vi "measure.vi"(8 "error in (no error)":errorcluster, 10 "Measure":bool, 11 "handle":i32) -> (0 "error out":errorcluster, 3 "state":i32)   [LabVIEW 2018]
uses:
  <userlib>/Gigahertz-Optik/GOMDTR9600/GOMDTR9600.lvlib
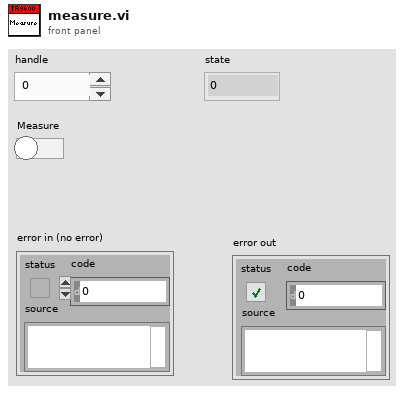
[diagram p1: front panel]
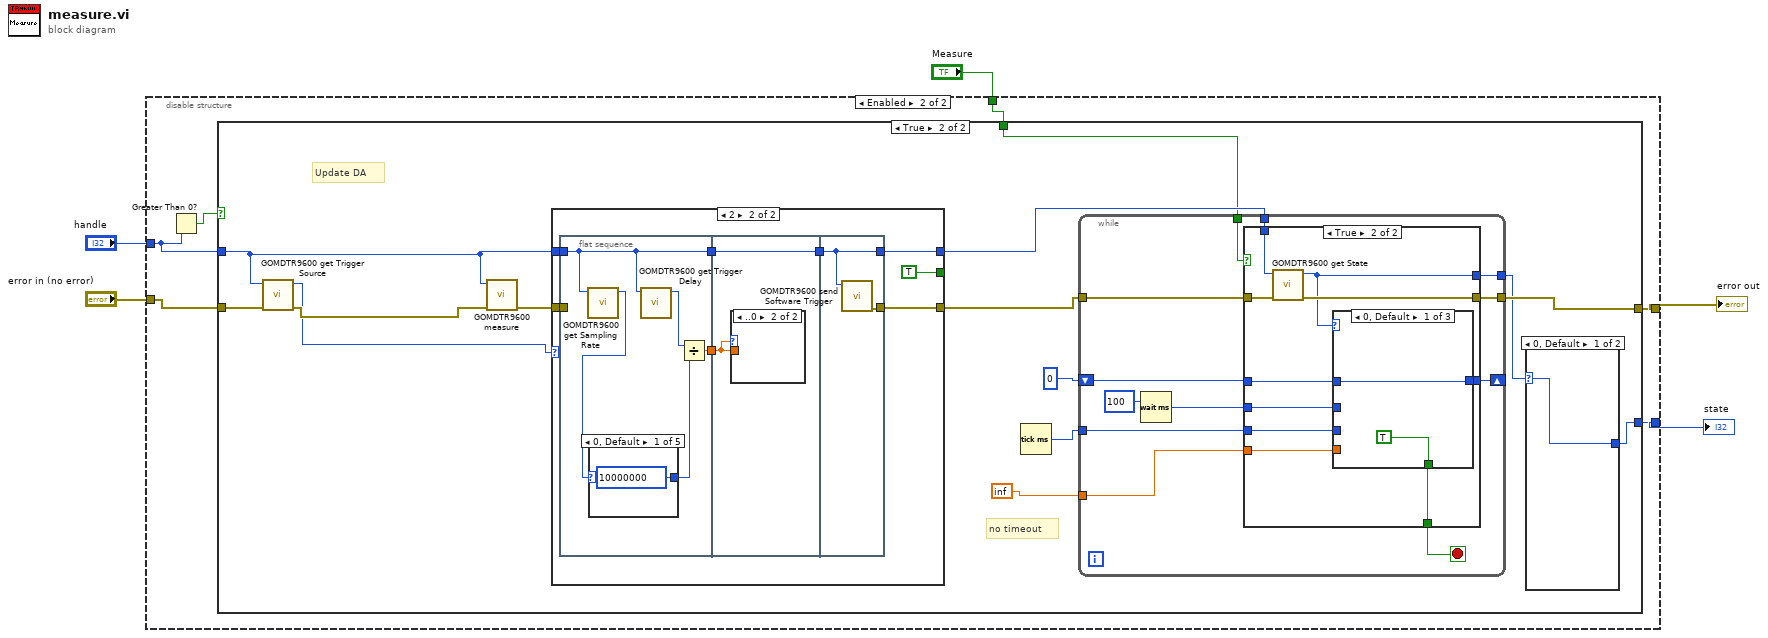
[diagram p0: block diagram]
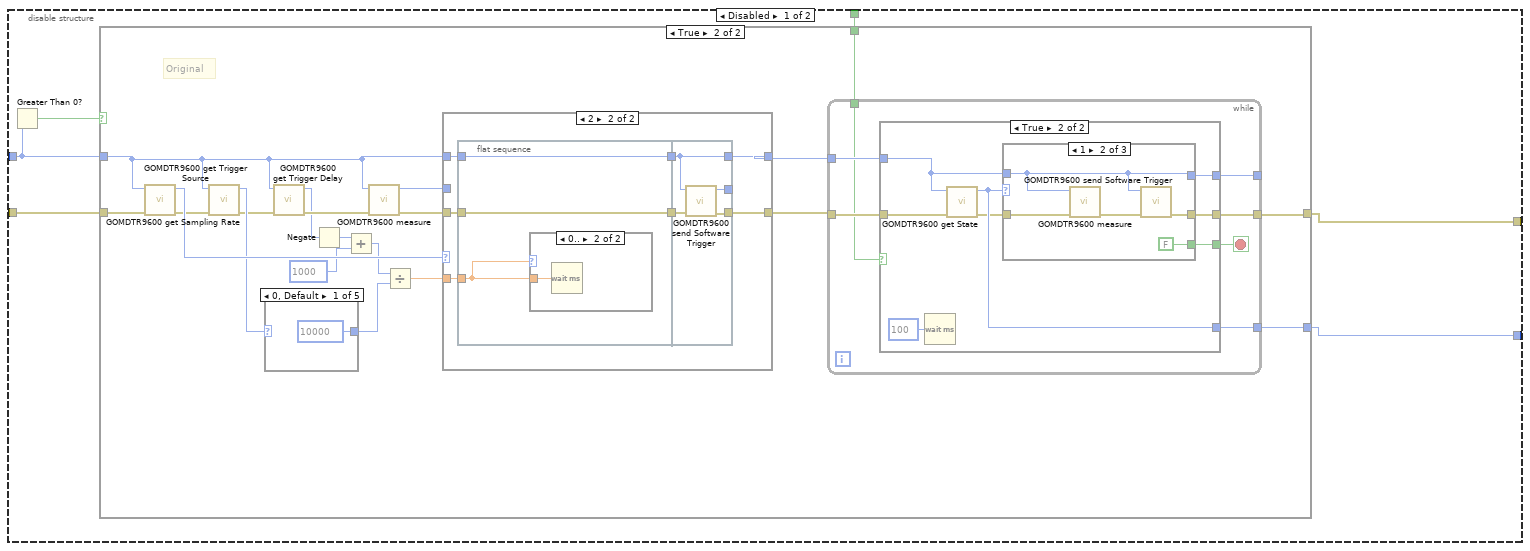
[diagram p2: hidden frame]
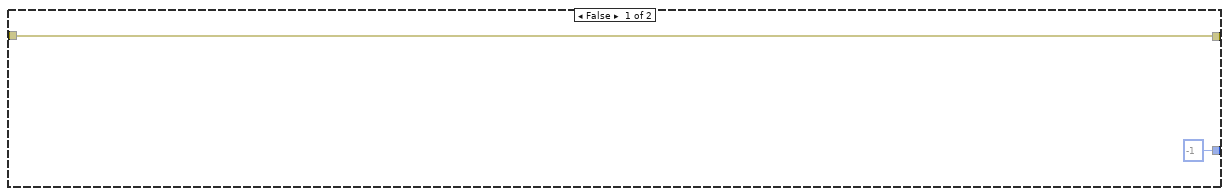
[diagram p3: hidden frame]
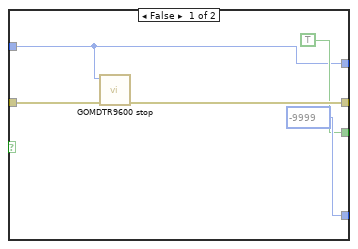
[diagram p4: hidden frame]
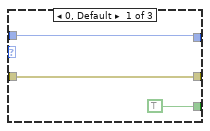
[diagram p5: hidden frame]
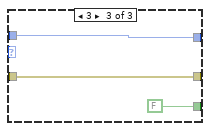
[diagram p6: hidden frame]
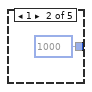
[diagram p7: hidden frame]
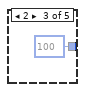
[diagram p8: hidden frame]
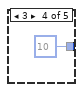
[diagram p9: hidden frame]
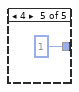
[diagram p10: hidden frame]
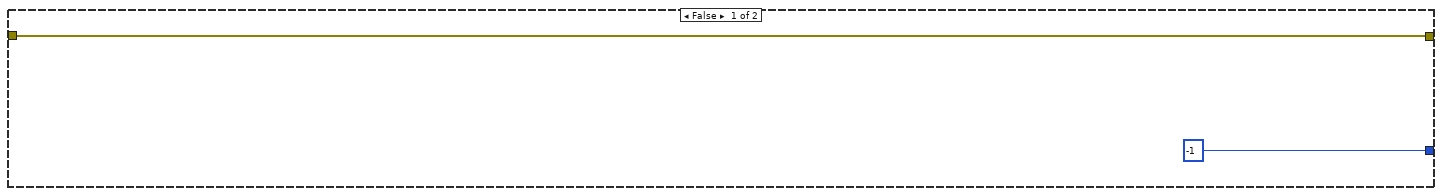
[diagram p13: hidden frame]
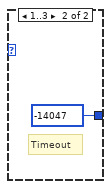
[diagram p14: hidden frame]
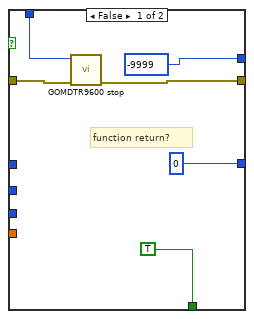
[diagram p15: hidden frame]
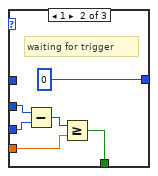
[diagram p16: hidden frame]
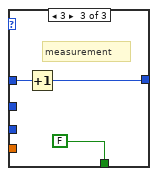
[diagram p17: hidden frame]
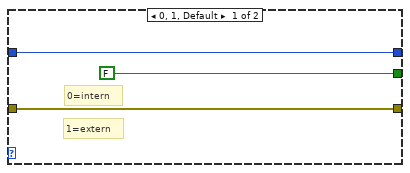
[diagram p18: hidden frame]
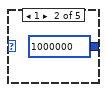
[diagram p19: hidden frame]
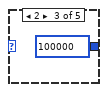
[diagram p20: hidden frame]
diagram:
  n1 = disable-structure shown="Enabled" {
    disable-tunnel: "error in (no error)" -> [w11 w87]
    disable-tunnel: "handle" -> [w10 w91]
    disable-tunnel: "Measure" -> [w9 w88]
    disable-tunnel: [w6 w90] -> w3
    disable-tunnel: [w7 w89] -> w2
    frame Disabled {
      n2 = Greater Than 0?(x=w10) -> (x > 0?=w8:bool)
      n3 = case shown="True" w8 {
        tunnel: w10 -> [_ w20]
        tunnel: w11 -> [w13 w19]
        tunnel: w9 -> [_ w16]
        tunnel: [w13 w15] -> w6
        tunnel: [-1 ("state") w14] -> w7
        frame False {
        }
        frame True {
          # "Original"
          n4 = call <userlib>:"GOMDTR9600 get Trigger Source.vi"("error in (no error)"=w19, "handle"=w20) -> ("error out"=w30:errorcluster, "value"=w32:i32)  [unwired: 7 in, 1 out]
          n5 = call <userlib>:"GOMDTR9600 get Sampling Rate.vi"("error in (no error)"=w30, "handle"=w20) -> ("error out"=w27:errorcluster, "value"=w29:i32)  [unwired: 7 in, 1 out]
          n6 = case shown="0, Default" w29 {
            tunnel: [10000 ("value") 1000 ("value") 100 ("value") 10 ("value") 1 ("value")] -> w28
            frame 0, Default {
            }
            frame 1 {
            }
            frame 2 {
            }
            frame 3 {
            }
            frame 4 {
            }
          }
          n7 = call <userlib>:"GOMDTR9600 get Trigger Delay.vi"("error in (no error)"=w27, "handle"=w20) -> ("error out"=w26:errorcluster, "value"=w25:i32)  [unwired: 7 in, 1 out]
          n8 = Negate(x=w25) -> (-x=w24:i32)
          n9 = Add(x=w24, y=1000) -> (x+y=w22:i32)
          n10 = call <userlib>:"GOMDTR9600 measure.vi"("error in (no error)"=w26, "handle"=w20) -> ("error out"=w33:errorcluster, "function return"=w31:i32)  [unwired: 8 in]
          n11 = Divide(x=w22, y=w28) -> (x/y=w21:dbl)
          n12 = case shown="2" w32 {
            tunnel: w33 -> [w71 w77]
            tunnel: [w71 w78] -> w17
            tunnel: w20 -> [w70 w76]
            tunnel: [w70 w75] -> w18
            tunnel: w31 -> [_ _]
            tunnel: w21 -> [_ w73]
            frame 0, 1, Default {
              # "1=extern"
              # "0=intern"
            }
            frame 2 {
              n13 = flat-sequence {
                tunnel: [w81] -> w74
                tunnel: w76 -> [w81]
                tunnel: w77 -> [w79]
                tunnel: w73 -> [w80]
                tunnel: [w79] -> w72
                tunnel: [w85] -> w78
                tunnel: w74 -> [w86]
                tunnel: [w86] -> w75
                tunnel: [w83] -> _
                tunnel: w72 -> [w84]
                frame #0 {
                  n14 = case shown="0.." w80 {
                    tunnel: w80 -> [_ w82]
                    frame Default {
                    }
                    frame 0.. {
                      n15 = Wait (ms)(milliseconds to wait=w82) -> ()  [unwired: 1 out]
                    }
                  }
                }
                frame #1 {
                  n16 = call <userlib>:"GOMDTR9600 send Software Trigger.vi"("error in (no error)"=w84, "handle"=w86) -> ("error out"=w85:errorcluster, "function return"=w83:i32)  [unwired: 8 in]
                }
              }
            }
          }
          n17 = while {
            tunnel: w17 -> [w40]
            tunnel: [w39] -> w15
            tunnel: [w38] -> w14
            tunnel: w18 -> [w37]
            tunnel: [w35] -> _
            tunnel: w16 -> [w34]
            stop <- w36 stop-if-true
            n18 = case shown="True" w34 {
              tunnel: w40 -> [w45 w53]
              tunnel: [w44 w48] -> w39
              tunnel: [-9999 ("function return") w52] -> w38
              tunnel: w37 -> [w41 w50]
              tunnel: [TRUE w51] -> w36
              tunnel: [w41 w46] -> w35
              frame False {
                n19 = call <userlib>:"GOMDTR9600 stop.vi"("error in (no error)"=w45, "handle"=w41) -> ("error out"=w44:errorcluster)  [unwired: 8 in, 1 out]
              }
              frame True {
                n20 = Wait (ms)(milliseconds to wait=u32 100) -> ()  [unwired: 1 out]
                n21 = call <userlib>:"GOMDTR9600 get State.vi"("error in (no error)"=w53, "handle"=w50) -> ("error out"=w49:errorcluster, "state"=w52:i32)  [unwired: 7 in, 1 out]
                n22 = case shown="1" w52 {
                  tunnel: [TRUE FALSE FALSE] -> w51
                  tunnel: w50 -> [w54 w59 w62]
                  tunnel: w49 -> [w55 w58 w63]
                  tunnel: [w55 w60 w63] -> w48
                  tunnel: [w54 w59 w62] -> w46
                  frame 0, Default {
                  }
                  frame 1 {
                    n23 = call <userlib>:"GOMDTR9600 measure.vi"("error in (no error)"=w58, "handle"=w59) -> ("error out"=w57:errorcluster)  [unwired: 8 in, 1 out]
                    n24 = call <userlib>:"GOMDTR9600 send Software Trigger.vi"("error in (no error)"=w57, "handle"=w59) -> ("error out"=w60:errorcluster)  [unwired: 8 in, 1 out]
                  }
                  frame 3 {
                  }
                }
              }
            }
          }
        }
      }
    }
    frame Enabled {
      n25 = Greater Than 0?(x=w91) -> (x > 0?=w92:bool)
      n26 = case shown="True" w92 {
        tunnel: w91 -> [_ w105]
        tunnel: w87 -> [w94 w108]
        tunnel: w88 -> [_ w95]
        tunnel: [w94 w98] -> w90
        tunnel: [-1 ("state") w96] -> w89
        frame False {
        }
        frame True {
          # "no timeout"
          # "Update DA"
          n27 = call <userlib>:"GOMDTR9600 get Trigger Source.vi"("error in (no error)"=w108, "handle"=w105) -> ("error out"=w107:errorcluster, "value"=w104:i32)  [unwired: 7 in, 1 out]
          n28 = call <userlib>:"GOMDTR9600 measure.vi"("error in (no error)"=w107, "handle"=w105) -> ("error out"=w106:errorcluster)  [unwired: 8 in, 1 out]
          n29 = case shown="2" w104 {
            tunnel: w106 -> [w152 w159]
            tunnel: [w152 w160] -> w103
            tunnel: w105 -> [w150 w157]
            tunnel: [FALSE ("Value") TRUE ("Value")] -> _
            tunnel: [w150 w156] -> w102
            frame 0, 1, Default {
              # "1=extern"
              # "0=intern"
            }
            frame 2 {
              n30 = flat-sequence {
                tunnel: w159 -> [_]
                tunnel: w157 -> [w165]
                tunnel: [w165] -> w155
                tunnel: [w163] -> w153
                tunnel: w155 -> [w172]
                tunnel: [w172] -> w154
                tunnel: w153 -> [w171]
                tunnel: [w174] -> w160
                tunnel: w154 -> [w175]
                tunnel: [w175] -> w156
                frame #0 {
                  n31 = call <userlib>:"GOMDTR9600 get Sampling Rate.vi"("handle"=w165) -> ("value"=w162:i32)  [unwired: 8 in, 2 out]
                  n32 = case shown="0, Default" w162 {
                    tunnel: [10000000 ("value") 1000000 ("value") 100000 ("value") 10000 ("value") 1000 ("value")] -> w161
                    frame 0, Default {
                    }
                    frame 1 {
                    }
                    frame 2 {
                    }
                    frame 3 {
                    }
                    frame 4 {
                    }
                  }
                  n33 = call <userlib>:"GOMDTR9600 get Trigger Delay.vi"("handle"=w165) -> ("value"=w164:i32)  [unwired: 8 in, 2 out]
                  n34 = Divide(x=w164, y=w161) -> (x/y=w163:dbl)
                }
                frame #1 {
                  n35 = case shown="..0" w171 {
                    tunnel: w171 -> [w173 _]
                    frame Default {
                      n36 = Wait (ms)(milliseconds to wait=w173) -> ()  [unwired: 1 out]
                    }
                    frame ..0 {
                    }
                  }
                }
                frame #2 {
                  n37 = call <userlib>:"GOMDTR9600 send Software Trigger.vi"("handle"=w175) -> ("error out"=w174:errorcluster)  [unwired: 9 in, 1 out]
                }
              }
            }
          }
          n38 = Tick Count (ms)() -> (millisecond timer value=w99:u32)
          n39 = while {
            tunnel: inf -> [w120]
            tunnel: w103 -> [w122]
            tunnel: [w121] -> w98
            tunnel: [w117] -> w97
            tunnel: w102 -> [w116]
            shift-right: [w113] -> _
            shift-left: 0 ("PBarValue") -> [w114]
            tunnel: w99 -> [w115]
            tunnel: w95 -> [w111]
            stop <- w112 stop-if-true
            n40 = Wait (ms)(milliseconds to wait=u32 100) -> (millisecond timer value=w118:u32)
            n41 = case shown="True" w111 {
              tunnel: w115 -> [_ w131]
              tunnel: w122 -> [w128 w138]
              tunnel: [w127 w137] -> w121
              tunnel: w120 -> [_ w130]
              tunnel: w118 -> [_ w132]
              tunnel: [-9999 ("function return") w135] -> w117
              tunnel: w116 -> [w125 w136]
              tunnel: w114 -> [_ w134]
              tunnel: [0 ("PBarValue") w133] -> w113
              tunnel: [TRUE w129] -> w112
              frame False {
                # "function return?"
                n42 = call <userlib>:"GOMDTR9600 stop.vi"("error in (no error)"=w128, "handle"=w125) -> ("error out"=w127:errorcluster)  [unwired: 8 in, 1 out]
              }
              frame True {
                n43 = call <userlib>:"GOMDTR9600 get State.vi"("error in (no error)"=w138, "handle"=w136) -> ("error out"=w137:errorcluster, "state"=w135:i32)  [unwired: 7 in, 1 out]
                n44 = case shown="0, Default" w135 {
                  tunnel: w134 -> [w140 _ w149]
                  tunnel: [w140 0 ("PBarValue") w148] -> w133
                  tunnel: w132 -> [_ w145 _]
                  tunnel: w131 -> [_ w144 _]
                  tunnel: w130 -> [_ w142 _]
                  tunnel: [TRUE w141 FALSE] -> w129
                  frame 0, Default {
                  }
                  frame 1 {
                    # "waiting for trigger"
                    n45 = Subtract(x=w145, y=w144) -> (x-y=w143:u32)
                    n46 = Greater Or Equal?(x=w143, y=w142) -> (x >= y?=w141:bool)
                  }
                  frame 3 {
                    # "measurement"
                    n47 = Increment(x=w149) -> (x+1=w148:i32)
                  }
                }
              }
            }
          }
          n48 = case shown="0, Default" w97 {
            selector: w97 -> [w109 _]
            tunnel: [w109 -14047 ("state")] -> w96
            frame 0, Default {
            }
            frame 1..3 {
              # "Timeout"
            }
          }
        }
      }
    }
  }
  "error out" <- w3
  "state" <- w2
